vi "OpenMainConsole.vi"(3 "Baxter in":T2) -> (1 "Baxter out":T2)   [LabVIEW 2013]
uses:
  _ROSControl.ctl
  _ROSDirection.ctl
panel:
  out "Execution:State":T1(ring)
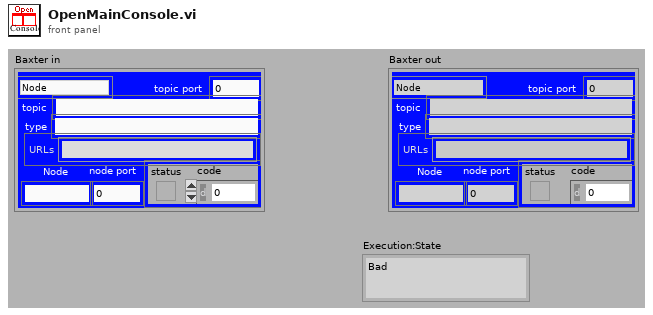
[diagram p1: front panel]
types:
  T1 = enum32{"Bad", "Idle", "Run top level", "Running"}
  T2 = typedef "_ROSControl.ctl" = cluster{"topic port":u16, "Node":string, "topic":string, "type":string, "node port":u32, "error ":errorcluster, "Direction":T3, "APIs":string[]}
  T3 = typedef "_ROSDirection.ctl" = enum16{"Node", "Publisher", "Subscriber", "Service Client"}
  T4 = enum32{"Invalid", "Standard", "Closed", "Hidden", "Minimized", "Maximized"}
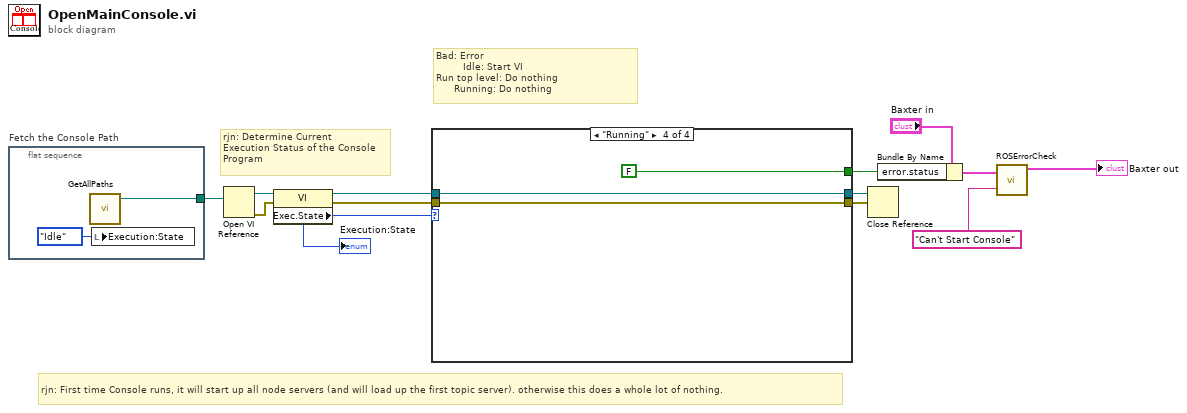
[diagram p0: block diagram]
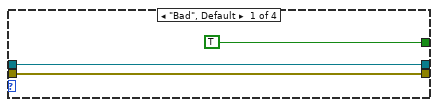
[diagram p2: hidden frame]
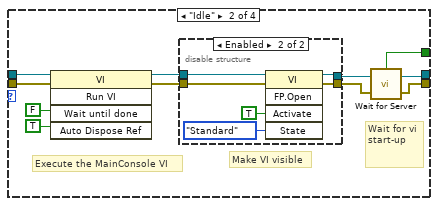
[diagram p3: hidden frame]
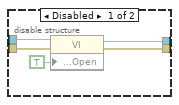
[diagram p4: hidden frame]
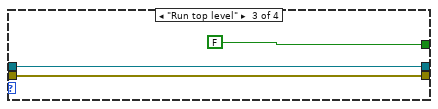
[diagram p5: hidden frame]
diagram:
  # "Bad: Error\n         Idle: Start VI\nRun top level: Do nothing\n      Running: Do nothing"
  # "rjn: Determine Current \nExecution Status of the Console\nProgram"
  # "rjn: First time Console runs, it will start up all node servers (and will load up the first topic server). otherwise this does a whole lot of nothing."
  n1 = flat-sequence "Fetch the Console Path" {
    tunnel: [w14] -> w10
    frame #0 {
      n2 = call "GetAllPaths.vi"() -> ("Console Path"=w14:path)  [unwired: 1 in, 2 out]
      n3 = local write "Execution:State"(T1."Idle" ("Execution:State")) -> ()
    }
  }
  n4 = Open VI Reference(vi path=w10) -> (vi reference=w11:refnum<vi>, error out=w9:errorcluster)  [unwired: 5 in]
  n5 = property class="VI"(reference=w11, error in=w9) -> (error out=w8:errorcluster, "Exec.State"=w7:T1)  [unwired: 1 out]
  "Execution:State" <- w7
  n6 = case shown="\"Running\"" w7 {
    tunnel: [w17 w22 w41 w44] -> w12
    tunnel: w11 -> [w17 w24 w41 w44]
    tunnel: [w16 w20 w40 w43] -> w6
    tunnel: w8 -> [w16 w26 w40 w43]
    tunnel: [TRUE ("Wait Until Done") w18 FALSE ("Wait Until Done") FALSE ("Wait Until Done")] -> w2
    frame "Bad", Default {
    }
    frame "Idle" {
      # "Wait for vi\nstart-up"
      # "Make VI visible"
      # "Execute the MainConsole VI"
      n7 = invoke class="VI" method="Run VI"(reference=w24, error in=w26, "Wait until done"=FALSE ("Wait Until Done"), "Auto Dispose Ref"=TRUE ("Wait Until Done")) -> (reference out=w19:refnum<vi>, error out=w25:errorcluster)  [unwired: 1 in, 3 out]
      n8 = disable-structure shown="Enabled" {
        disable-tunnel: w25 -> [w32 w36]
        disable-tunnel: [w31 w35] -> w23
        disable-tunnel: [w30 w34] -> w21
        disable-tunnel: w19 -> [w29 w37]
        frame Disabled {
          n9 = property class="VI"(reference=w29, error in=w32, "Front Panel.Open"=TRUE ("Wait Until Done")) -> (reference out=w31:refnum<vi>, error out=w30:errorcluster)
        }
        frame Enabled {
          n10 = invoke class="VI" method="FP.Open"(reference=w37, error in=w36, "Activate"=TRUE ("Activate?"), "State"=T4."Standard") -> (reference out=w35:refnum<vi>, error out=w34:errorcluster)  [unwired: 1 in, 3 out]
        }
      }
      n11 = call "Wait for Server.vi"("error in"=w21, "vi reference in"=w23) -> ("error out"=w20:errorcluster, "Error?"=w18:bool, "vi reference out"=w22:refnum<vi>)
    }
    frame "Run top level" {
    }
    frame "Running" {
    }
  }
  n12 = Close Reference(reference=w12, error in (no error)=w6) -> ()  [unwired: 1 out]
  n13 = Bundle By Name(cluster="Baxter in", "error.status"=w2) -> (w1:T2)
  n14 = call "ROSErrorCheck.vi"("message"="Can't Start Console", "ROS in"=w1) -> ("ROS out"=→"Baxter out":T2)  [unwired: 1 in]
